vi "extract_phase_from_transmission.vi"(9 "Mask B Calibration Path":path=path "G:/My Drive/ansom/Data/THz 1/pulse shaping/SLM Calibration 09March22/Final 1D Mask B.txt", 10 "Mask A Calibration Path":path=path "G:/My Drive/ansom/Data/THz 1/pulse shaping/SLM Calibration 09March22/Final 1D Mask A.txt", 11 "Pixel number":dbl=250.0 format="%#_13g") -> (2 "Mask B Phase":cluster{"Ramp Pattern":dbl[], "phase out":dbl[]}(graph), 3 "Mask A Phase":cluster{"Ramp Pattern":dbl[], "phase out":dbl[]}(graph))   [LabVIEW 2019]
uses:
  <vilib>/Analysis/1siggen.llb/Ramp Pattern by Delta.vi
  <vilib>/Analysis/NI_AALBase.lvlib
panel:
  out "Mask A Transmission":cluster{"Ramp Pattern":dbl[], "phase out":dbl[]}(graph)
  out "Mask B Transmission":cluster{"Ramp Pattern":dbl[], "phase out":dbl[]}(graph)
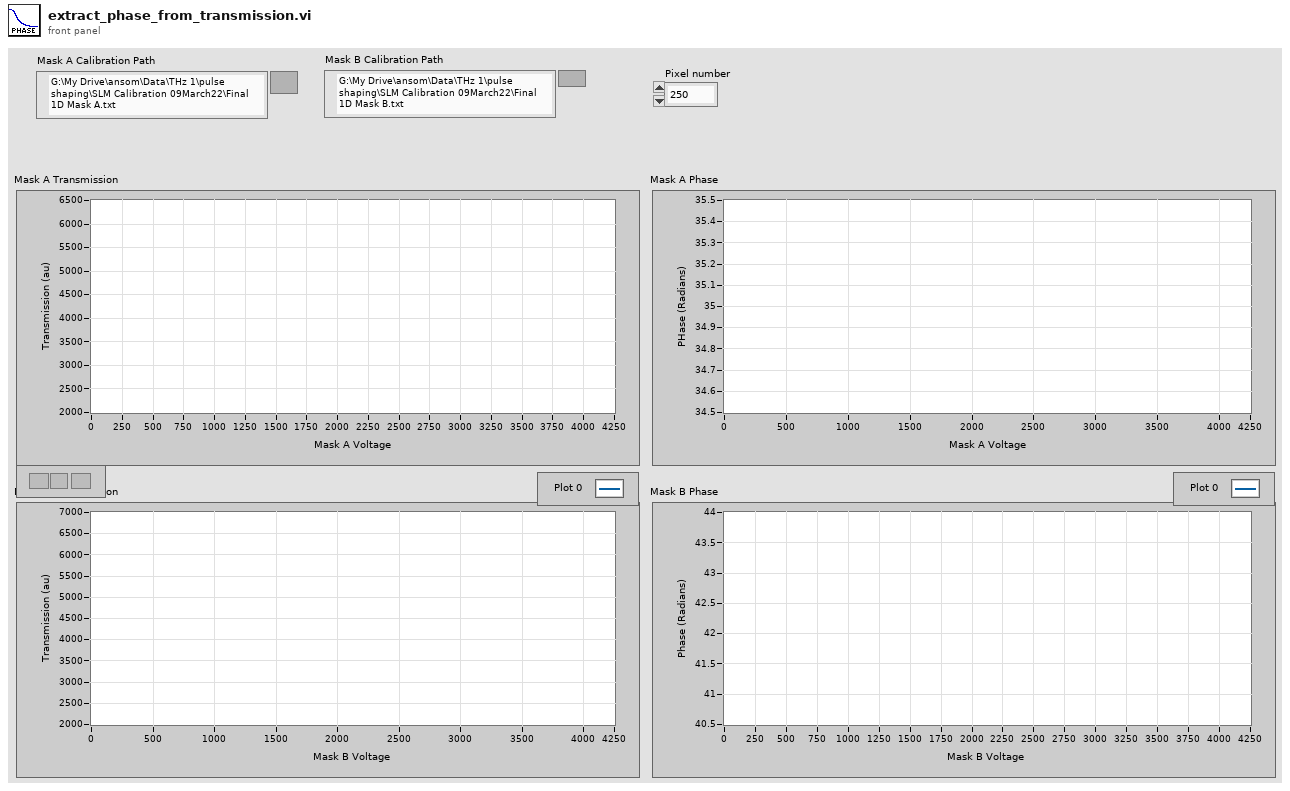
[diagram p1: front panel]
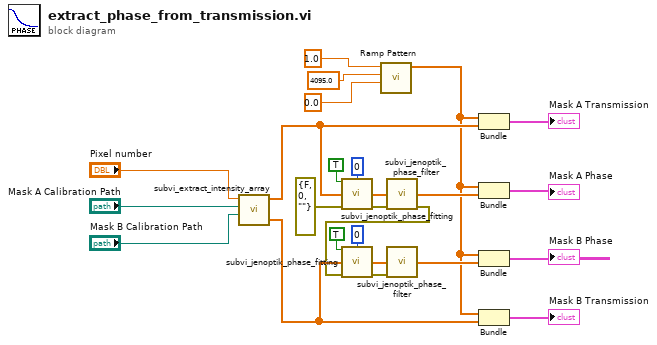
[diagram p0: block diagram]
diagram:
  n1 = call "subvi_extract_intensity_array.vi"("Mask B Path"="Mask B Calibration Path", "Mask A Path"="Mask A Calibration Path", "Pixel"="Pixel number") -> ("Mask B Y"=w25:dbl[], "Mask A Y"=w24:dbl[])  [unwired: 7 in]
  n2 = call "subvi_jenoptik_phase_fitting.vi"("allow last extremum to be minimum?"=TRUE, "algorithm"=0, "intensity"=w24, "error in (no error)"=errorcluster {"status"=FALSE, "code"=0, "source"=""}) -> ("phase"=w11:dbl[], "error out"=w9:errorcluster)  [unwired: 10 in]
  n3 = call-poly <vilib>:"Ramp Pattern.vi"("start"=0.0, "end"=4095.0, "delta"=1.0) -> ("Ramp Pattern"=w7:dbl[])  [unwired: 6 in, 2 out]
  n4 = call "subvi_jenoptik_phase_filter.vi"("phase in"=w11, "error in (no error)"=w9) -> ("phase out"=w10:dbl[], "error out"=w8:errorcluster)  [unwired: 12 in]
  n5 = call "subvi_jenoptik_phase_fitting.vi"("allow last extremum to be minimum?"=TRUE, "algorithm"=0, "intensity"=w25, "error in (no error)"=w8) -> ("phase"=w13:dbl[], "error out"=w12:errorcluster)  [unwired: 10 in]
  n6 = call "subvi_jenoptik_phase_filter.vi"("phase in"=w13, "error in (no error)"=w12) -> ("phase out"=w14:dbl[])  [unwired: 12 in, 1 out]
  n7 = Bundle("Ramp Pattern"=w7, "Mask A Y"=w24) -> (→"Mask A Transmission":cluster{"Ramp Pattern":dbl[], "Mask A Y":dbl[]})  [unwired: 1 in]
  n8 = Bundle("Ramp Pattern"=w7, "phase out"=w10) -> (→"Mask A Phase":cluster{"Ramp Pattern":dbl[], "phase out":dbl[]})  [unwired: 1 in]
  n9 = Bundle("Ramp Pattern"=w7, "phase out"=w14) -> (→"Mask B Phase":cluster{"Ramp Pattern":dbl[], "phase out":dbl[]})  [unwired: 1 in]
  n10 = Bundle("Ramp Pattern"=w7, "Mask B Y"=w25) -> (→"Mask B Transmission":cluster{"Ramp Pattern":dbl[], "Mask B Y":dbl[]})  [unwired: 1 in]
